vi "DAQ-AOtest.vi"() -> ()   [LabVIEW 2020]
uses:
  <vilib>/DAQmx/write.llb/DAQmx Write.vi
  <vilib>/DAQmx/write.llb/DAQmx Write (Analog 1D Wfm NChan NSamp).vi
  <vilib>/DAQmx/create/channels.llb/DAQmx Create Channel (AO-Voltage-Basic).vi
  <vilib>/DAQmx/configure/timing.llb/DAQmx Timing (Sample Clock).vi
  <vilib>/DAQmx/miscellaneous.llb/DAQmx Fill In Error Info.vi
  <resource>/objmgr/daqmx.rc
panel:
  out "error out":errorcluster
  in  "error in":errorcluster
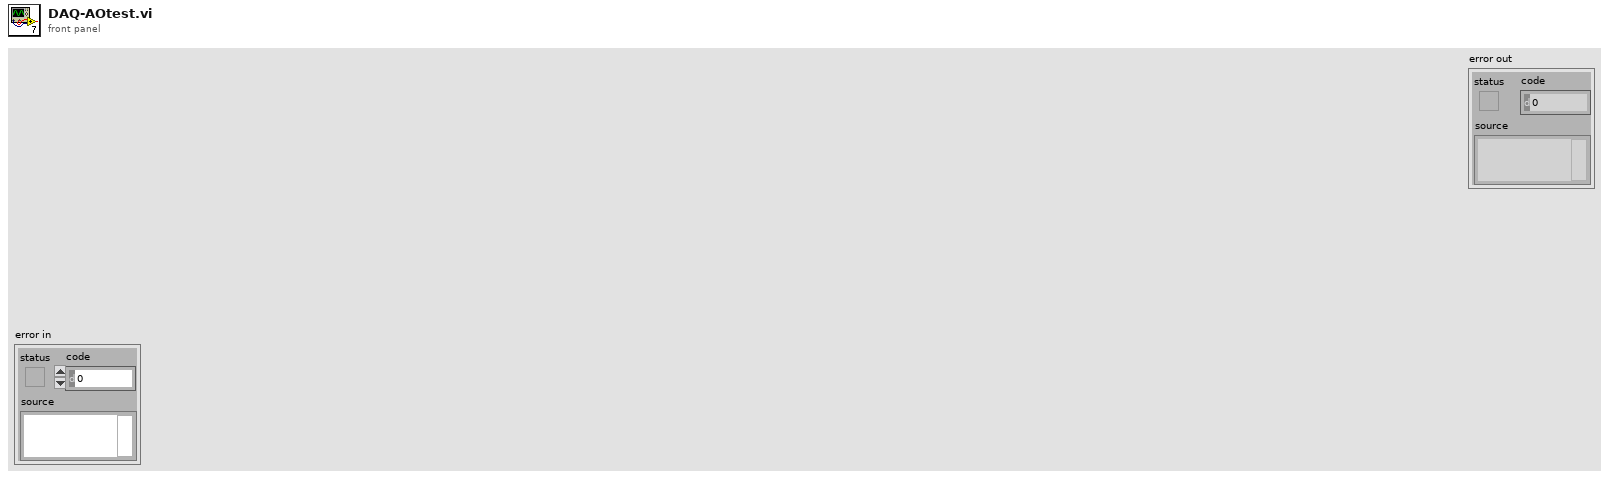
[diagram p1: front panel]
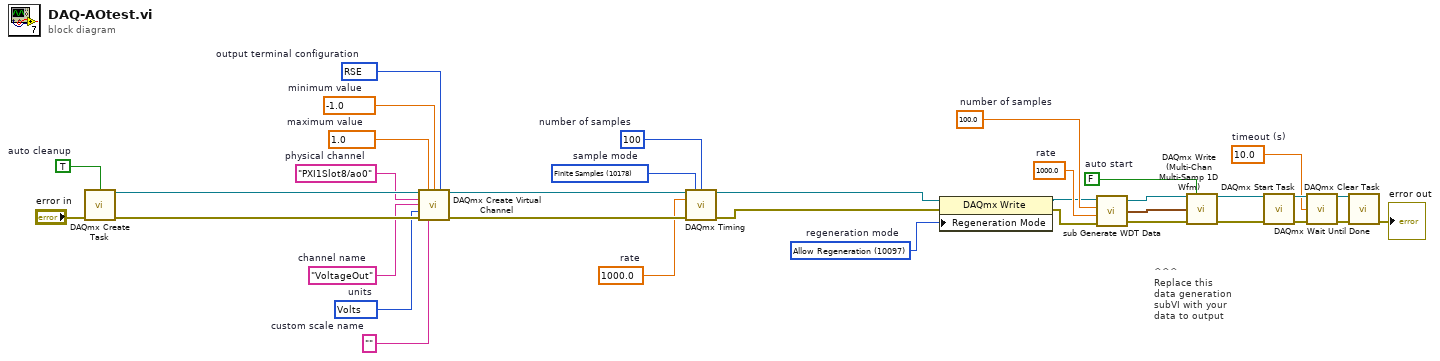
[diagram p0: block diagram]
diagram:
  w4 = 10097 items=["Allow Regeneration"=10097, "Do Not Allow Regeneration"=10158]  # regeneration mode
  w6 = 10178 items=["Finite Samples"=10178, "Continuous Samples"=10123, "Hardware Timed Single Point"=12522]  # sample mode
  w7 = 100  # number of samples
  w8 = 1000.0  # rate
  w11 = 10083 items=["Default"=-1, "RSE"=10083, "Differential"=10106, "Pseudodifferential"=12529]  # output terminal configuration
  w12 = 10348 items=["Volts"=10348, "From Custom Scale"=10065]  # units
  w13 = "VoltageOut"  # channel name
  w15 = ""  # custom scale name
  w16 = -1.0  # minimum value
  w17 = 1.0  # maximum value
  w18 = "PXI1Slot8/ao0"  # physical channel
  w20 = TRUE  # auto cleanup
  w26 = 10.0  # timeout (s)
  w30 = 1000.0  # rate
  w31 = 100.0  # number of samples
  w35 = FALSE  # auto start
  # "^^^\nReplace this\ndata generation\nsubVI with your\ndata to output"
  n1 = call <vilib>:"DAQmx Create Task.vi"("auto cleanup"=w20, "error in"="error in") -> ("task out"=w19:refnum<k21>, "error out"=w21:errorcluster)  [unwired: 12 in]
  n2 = call-poly <vilib>:"DAQmx Create Virtual Channel.vi"("task in"=w19, "maximum value"=w17, "minimum value"=w16, "output terminal configuration"=w11, "physical channels"=w18, "name to assign"=w13, "units"=w12, "error in"=w21, "custom scale name"=w15) -> ("task out"=w9:refnum<k21>, "error out"=w14:errorcluster)  [unwired: 5 in]
  n3 = call-poly <vilib>:"DAQmx Timing.vi"("task/channels in"=w9, "sample mode"=w6, "samples per channel"=w7, "rate"=w8, "error in"=w14) -> ("task out"=w5:refnum<k21>, "error out"=w10:errorcluster)  [unwired: 9 in]
  n4 = property class="DAQmx Write"(reference=w5, error in=w10, "Regeneration Mode"=w4) -> (reference out=w2:refnum<k21>, error out=w3:errorcluster)
  n5 = call <vilib>:"sub Generate WDT Data.vi"("task in"=w2, "number of samples"=w31, "update rate"=w30, "error in"=w3) -> ("task out"=w33:refnum<k21>, "Data"=w32:waveform(dbl)[], "error out"=w34:errorcluster)  [unwired: 1 in]
  n6 = call-poly "DAQmx Write (Multi-Chan Multi-Samp 1D Wfm).vi"("task/channels in"=w33, "auto start"=w35, "data"=w32, "error in"=w34) -> ("task out"=w25:refnum<k21>, "error out"=w24:errorcluster)  [unwired: 9 in, 1 out]
  n7 = call <vilib>:"DAQmx Start Task.vi"("task/channels in"=w25, "error in"=w24) -> ("task out"=w29:refnum<k21>, "error out"=w28:errorcluster)  [unwired: 12 in]
  n8 = call <vilib>:"DAQmx Wait Until Done.vi"("task/channels in"=w29, "timeout (sec)"=w26, "error in"=w28) -> ("task out"=w23:refnum<k21>, "error out"=w27:errorcluster)  [unwired: 11 in]
  n9 = call <vilib>:"DAQmx Clear Task.vi"("task in"=w23, "error in"=w27) -> ("error out"=→"error out":errorcluster)  [unwired: 13 in]
